vi "Request Synchronous Data (Boolean).vi"(6 "Ignore Past Updates? (F)":bool, 7 "Timeout In ms (-1)":i32=-1, 8 "error in (no error)":errorcluster, 9 "Type (Boolean)":bool, 10 "Datum Name":string, 11 "IModel In":refnum<class "IModel.lvclass">) -> (0 "error out":errorcluster, 1 "timed out?":bool, 2 "Data (Boolean)":bool, 4 "Publication Time":timestamp)   [LabVIEW 2017, in "IModel.lvlib" / "IModel.lvclass"]
doc: "<License>\nCopyright © 2017 Composed Systems, LLC | All rights reserved\nwww.composed.io\n\nAuthor: Ethan Stern <ethan.stern@composed.io>\n\nThis software is provided \"AS IS\" WITHOUT WARRANTIES, either express or implied, AND IS FOR EDUCATIONAL PURPOSES ONLY.\n</License>"
uses:
  IModel.lvclass
  C:/Git/mva-framework/Framework/IObserver/IObserver/IObserver.lvclass
  IObserver/IObserver/IObserver.lvclass/IObserver.ctl
  SubscriptionPolicy/OneShotSubscription/OneShotSubscription.lvclass/OneShotSubscription.ctl
  Transport/QueueTransport/QueueTransport.lvclass/QueueTransport.ctl
  IMediator/SubscriptionRequest/SubscriptionRequest.lvclass/SubscriptionRequest.ctl
  AbstractMessages/PreAddressedMsg/PreAddressedMsg.lvclass/PreAddressedMsg.ctl
  IMediator/IMediator Messages/Subscribe Msg/Subscribe Msg.lvclass/Subscribe Msg.ctl
  <vilib>/ActorFramework/Message Enqueuer/Message Enqueuer.lvclass/Message Enqueuer.ctl
  Transport/QueueTransport/New Queue Transport.vi
  IMediator/SubscriptionRequest/Pack Subscription Request.vi
  SubscriptionPolicy/OneShotSubscription/New One-Shot Subscription.vi
  IMediator/IMediator Messages/Subscribe Msg/Send Pre-Addressed Subscribe.vi
  Transport/QueueTransport/Dequeue Transport Element.vi
  IObserver/IObserver/Read Subscribe Msg.vi
  <vilib>/ActorFramework/Message Enqueuer/Enqueue.vi
  AbstractMessages/PreAddressedMsg/Read Return Address.vi
  Transport/QueueTransport/QueueTransport.lvclass
  C:/Git/mva-framework/Framework/IMediator/ITransport/ITransport.lvclass
  SubscriptionPolicy/OneShotSubscription/OneShotSubscription.lvclass
  C:/Git/mva-framework/Framework/IMediator/ISubscriptionPolicy/ISubscriptionPolicy.lvclass
  IMediator/IMediator Messages/Subscribe Msg/Subscribe Msg.lvclass
  C:/Git/mva-framework/Framework/AbstractMessages/PreAddressedMsg/PreAddressedMsg.lvclass
  C:/Program Files (x86)/National Instruments/LabVIEW 2017/vi.lib/ActorFramework/Message/Message.lvclass
  <vilib>/Utility/error.llb/Error Cluster From Error Code.vi
  <vilib>/ActorFramework/Message Priority Queue/Priority Enqueue.vi
  IMediator/ISubscriptionPolicy/Open Subscription Policy.vi
  IMediator/SubscriptionRequest/SubscriptionRequest.lvclass
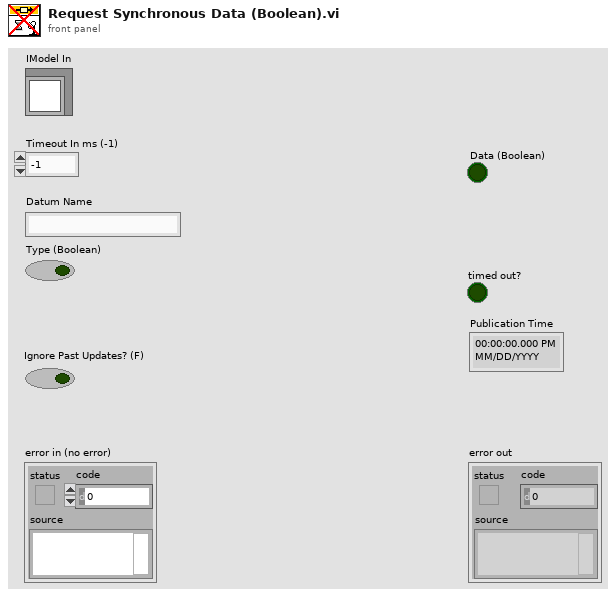
[diagram p1: front panel]
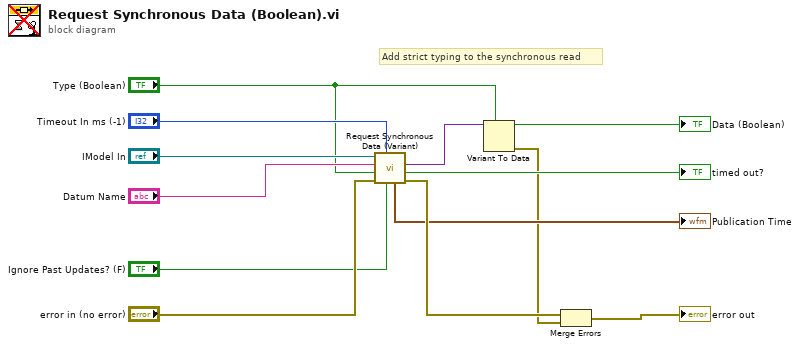
[diagram p0: block diagram]
diagram:
  # "Add strict typing to the synchronous read"
  n1 = call "Request Synchronous Data (Variant).vi"("Ignore Past Updates? (F)"="Ignore Past Updates? (F)", "Timeout In ms (-1)"="Timeout In ms (-1)", "error in (no error)"="error in (no error)", "Type"="Type (Boolean)", "Datum Name"="Datum Name", "IModel In"="IModel In") -> ("error out"=w10:errorcluster, "timed out?"=→"timed out?":bool, "Data"=w6:variant, "Publication Time"=→"Publication Time":timestamp)  [unwired: 2 in]
  n2 = Variant To Data(type="Type (Boolean)", Variant=w6) -> (data=→"Data (Boolean)":bool, error out=w1:errorcluster)  [unwired: 1 in]
  n3 = Merge Errors(w10, w1) -> (→"error out":errorcluster)
